vi "WPI_AnalogModuleGetVoltage.vi"(8 "error in (no error)":errorcluster, 10 "Channel":T2, 11 "AnalogModuleDevRef":T1) -> (0 "error out":errorcluster, 2 "Voltage":dbl, 3 "AnalogModuleDevRef":T1)   [LabVIEW 2017]
doc: "This software is licensed. Open the labview\\readme\\WPI Robotics Library Open Source License.txt file for more information."
uses:
  <vilib>/Rock Robotics/SystemInterfaces/AI/FPGA_AIChannel.ctl
  <vilib>/Rock Robotics/WPI/AnalogModule/WPI_AnalogModuleDevStatus.ctl
  <vilib>/Rock Robotics/SystemInterfaces/System/FPGA_SystemGet.vi
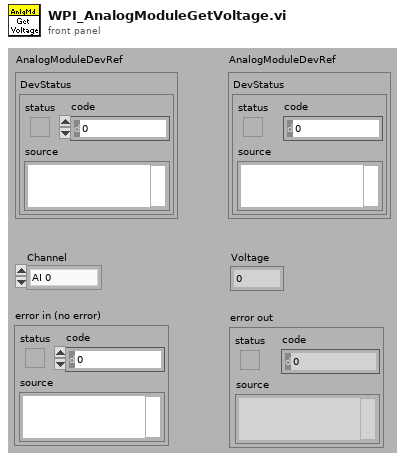
[diagram p1: front panel]
types:
  T1 = typedef "WPI_AnalogModuleDevStatus.ctl" = cluster{"DevStatus":errorcluster}
  T2 = typedef "FPGA_AIChannel.ctl" = enum8{"AI 0", "AI 1", "AI 2", "AI 3", "AI MXP 0", "AI MXP 1", "AI MXP 2", "AI MXP 3", "Invalid"}
  T3 = typedef "FPGA_AIDevRef.ctl" = cluster{"DevStatus":errorcluster}
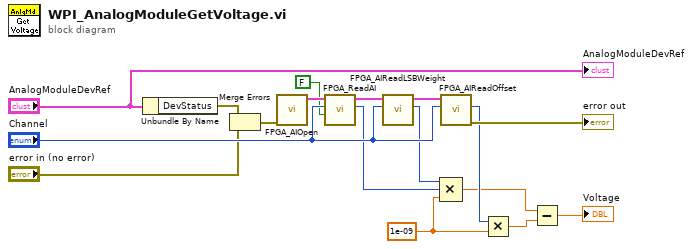
[diagram p0: block diagram]
diagram:
  w8 = 1e-09 ("y")
  n1 = Unbundle By Name("AnalogModuleDevRef") -> ("DevStatus"=w5:errorcluster)
  n2 = Merge Errors(w5, "error in (no error)") -> (w2:errorcluster)
  n3 = call <vilib>:"FPGA_AIOpen.vi"("error in (no error)"=w2) -> ("AI Reference out"=w11:T3)  [unwired: 2 in, 8 out]
  n4 = call <vilib>:"FPGA_ReadAI.vi"("average?"=FALSE, "Channel"="Channel", "AI Reference"=w11) -> ("Value"=w9:i32, "AI Reference"=w10:T3)  [unwired: 1 in, 6 out]
  n5 = call <vilib>:"FPGA_AIReadLSBWeight.vi"("Channel"="Channel", "AI Reference"=w10) -> ("LSBWeight"=w4:u32, "AI Reference"=w14:T3)  [unwired: 1 in, 7 out]
  n6 = Compound Arithmetic op=MULTIPLY(w4, w9, w8) -> (w7:dbl)
  n7 = call <vilib>:"FPGA_AIReadOffset.vi"("Channel"="Channel", "AI Reference"=w14) -> ("error out"=→"error out":errorcluster, "Offset"=w13:i32)  [unwired: 1 in, 7 out]
  n8 = Multiply(x=w13, y=w8) -> (x*y=w12:dbl)
  n9 = Subtract(x=w7, y=w12) -> (x-y=→"Voltage":dbl)
  "AnalogModuleDevRef" <- "AnalogModuleDevRef"
